vi "Get Config File Path.vi"(8 "error in (no error)":errorcluster, 11 "Base Path":path) -> (0 "error out":errorcluster, 3 "XML File Path":path)   [LabVIEW 2013, in "Cal Inst.lvlib" / "Cal Inst Settings.lvlib"]
doc: "Get the path to the Settings XML file. This is done using the Application Directory function. For more information on how Application Directory calculates its path, right-click the function and choose Help."
uses:
  Cal Inst Settings.lvlib
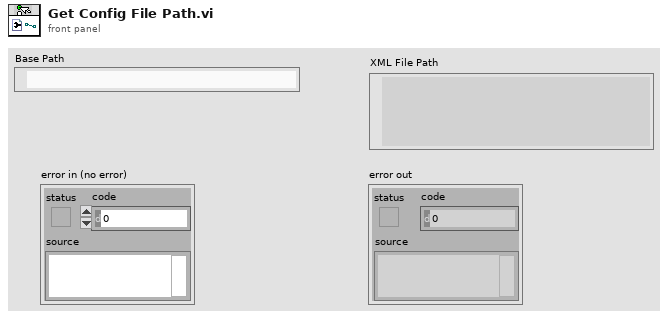
[diagram p1: front panel]
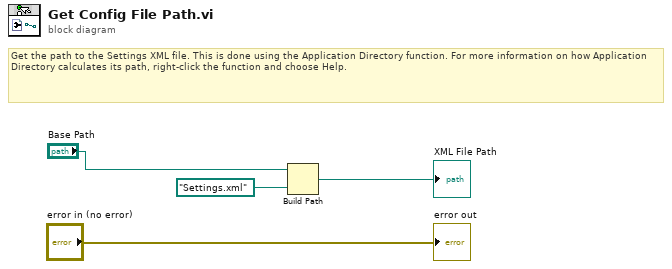
[diagram p0: block diagram]
diagram:
  # "Get the path to the Settings XML file. This is done using the Application Directory function. For more information on how Application Directory calculates its path, right-click the function and choose Help."
  n1 = Build Path(base path="Base Path", name or relative path=path "Settings.xml" ("string")) -> (appended path=→"XML File Path":path)
  "error out" <- "error in (no error)"
